vi "TSP_GA Solver.vi"(1 "pop_size":dbl=100.0, 2 "Number of Iterative":dbl) -> ()   [LabVIEW 2016]
panel:
  out "opt_rte":dbl[](array[numeric])
  out "Numeric":i32
  out "error out":errorcluster
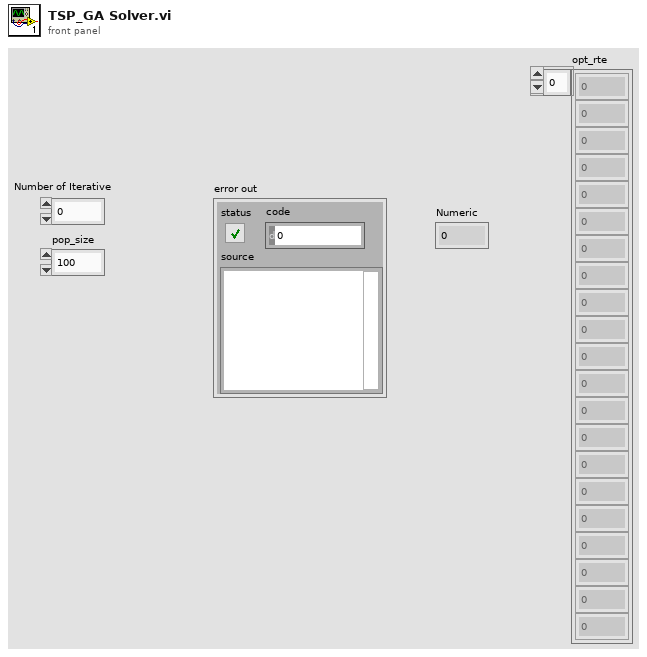
[diagram p1: front panel]
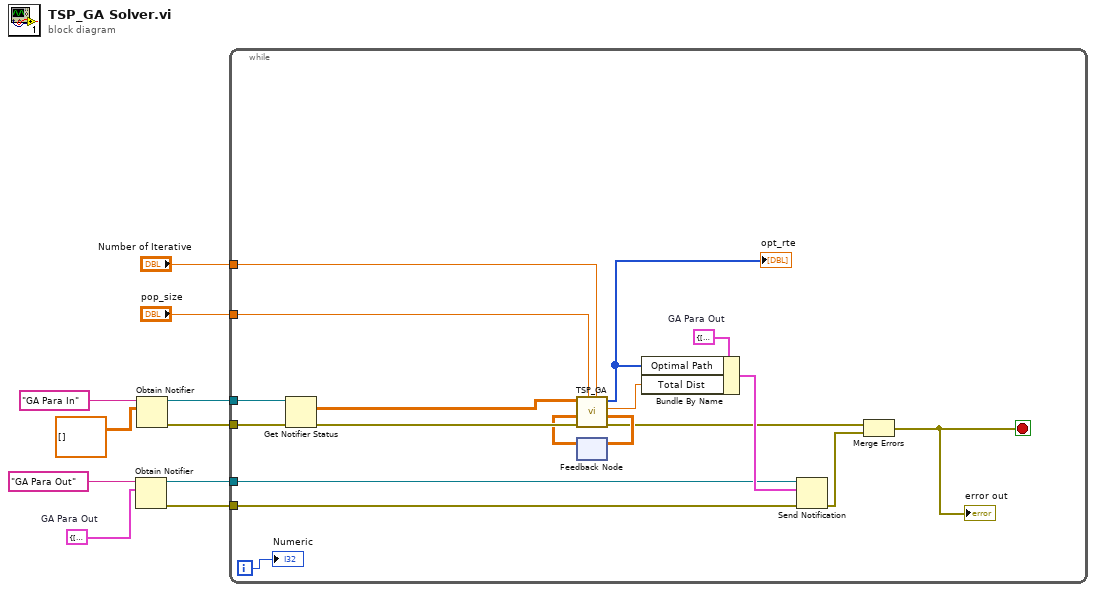
[diagram p0: block diagram]
diagram:
  w4 = cluster{"Optimal Path":dbl[], "Total Dist":dbl} {"Optimal Path"=[], "Total Dist"=0.0}  # GA Para Out
  n1 = Obtain Notifier(name (unnamed)="GA Para Out", notification data type=w4) -> (notifier out=w3:refnum<notifier>, error out=w2:errorcluster)  [unwired: 2 in, 1 out]
  n2 = Obtain Notifier(name (unnamed)="GA Para In", notification data type=dbl[][] []) -> (notifier out=w6:refnum<notifier>, error out=w7:errorcluster)  [unwired: 2 in, 1 out]
  n3 = while {
    tunnel: w6 -> [w28]
    tunnel: w7 -> [w27]
    tunnel: "pop_size" -> [w21]
    tunnel: "Number of Iterative" -> [w20]
    tunnel: w3 -> [w16]
    tunnel: w2 -> [w15]
    i -> [w19]
    stop <- w12 stop-if-true
    w17 = cluster{"Optimal Path":dbl[], "Total Dist":dbl} {"Optimal Path"=[], "Total Dist"=0.0}  # GA Para Out
    n4 = Get Notifier Status(notifier=w28, error in (no error)=w27) -> (current notification=w11:dbl[][], error out=w26:errorcluster)  [unwired: 3 out]
    n5 = feedback #1() -> (w22:dbl[][])  [unwired: 1 in]
    n6 = call "TSP_GA.vi"("Number of Iterative"=w20, "pop_size"=w21, "error in"=w26, "Pop in"=w22, "xy"=w11) -> ("error out"=w13:errorcluster, "pop out"=w23:dbl[][], "min dist"=w24:dbl, "opt_rte"=w25:i16[])  [unwired: 2 in, 1 out]
    "opt_rte" <- w25
    n7 = feedback-in #1(w23) -> ()
    n8 = Bundle By Name(cluster=w17, "Optimal Path"=w25, "Total Dist"=w24) -> (w18:cluster{"Optimal Path":dbl[], "Total Dist":dbl})
    n9 = Send Notification(notification=w18, notifier=w16, error in (no error)=w15) -> (error out=w14:errorcluster)  [unwired: 1 out]
    n10 = Merge Errors(w13, w14) -> (w12:errorcluster)
    "error out" <- w12
    "Numeric" <- w19
  }
